vi "Read ERD Multiple Message Example.vi"(0 "GEA2 Reference In":refnum<k24>, 1 "Retry Count":i32=2, 2 "Read Timeout (ms)":u32=500, 5 "GEA Inputs":T3 {"Destination" format="%.0x"; "Source" format="%.0x"}, 11 "Error In":errorcluster, 12 "#ERDs per message":i32=1 min=1 step=1, 13 "Verify ERD Response?":bool=TRUE, 14 "Low Level Retry Count":u8=5 min=1 step=1) -> (4 "GEA2 Reference Out":refnum<k24>, 6 "Board ID":string, 8 "Raw Data Out":string[](array[string]), 15 "Error Out":errorcluster)   [LabVIEW 2016]
doc: "This is an example of how to use the GEA2 Read ERD multi-message VI. This VI splits up multiple ERD read requests into the number of messages you specify."
uses:
  Q:/Common/DLLs/GEA3/GeaCommunication.dll
  DLLs/GEA3/GeaCommunication.dll
  LabVIEW_GEA2_Toolkit.lvlibp/type defs/Source_Destination.ctl
  LabVIEW_GEA2_Toolkit.lvlibp/type defs/ERD Read Data In.ctl
  LabVIEW_GEA2_Toolkit.lvlibp/type defs/Data Type.ctl
  LabVIEW_GEA2_Toolkit.lvlibp
panel:
  in  "Read ERD List":T1[](array[typedef]) {"ERD Number" format="%.0x"}
  in  "Standalone?":bool=TRUE
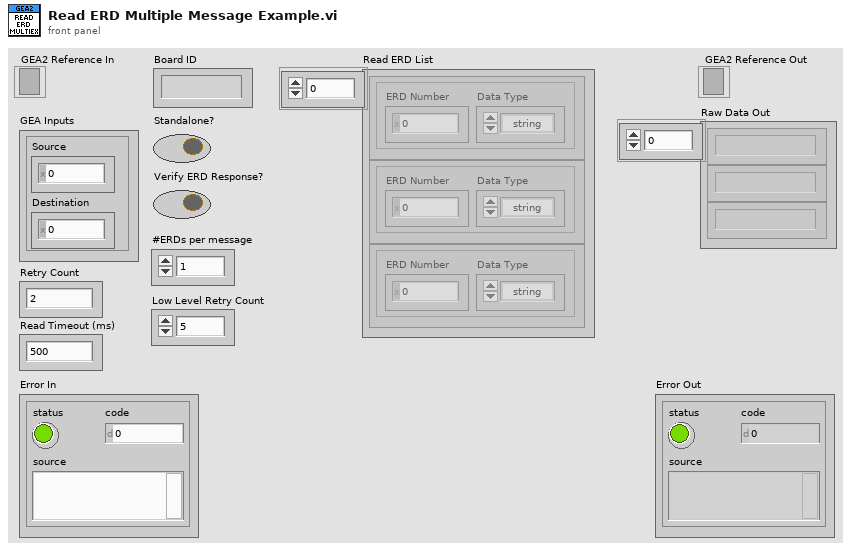
[diagram p1: front panel]
types:
  T1 = typedef "LabVIEW_GEA2_Toolkit.lvlibp/ERD Read Data In.ctl" = cluster{"ERD Number":u16, "Data Type":T2}
  T2 = typedef "LabVIEW_GEA2_Toolkit.lvlibp/Data Type.ctl" = enum16{"string", "boolean", "uint8_t", "uint16_t", "uint32_t", "uint64_t", "int8_t", "int16_t", "int32_t", "int64_t"}
  T3 = typedef "LabVIEW_GEA2_Toolkit.lvlibp/Source_Destination.ctl" = cluster{"Source":u8, "Destination":u8}
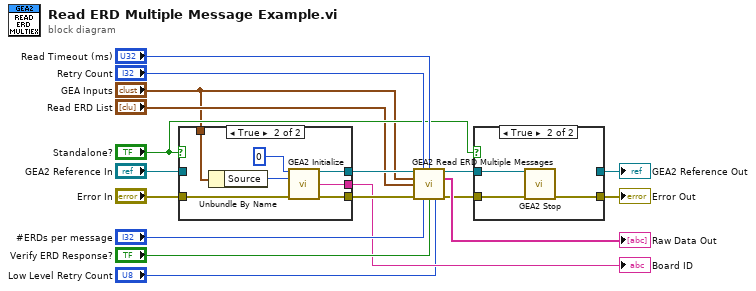
[diagram p0: block diagram]
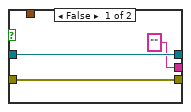
[diagram p3: hidden frame]
diagram:
  n1 = case shown="True" "Standalone?" {
    tunnel: [w20 w28] -> w15
    tunnel: "Error In" -> [w20 w27]
    tunnel: [w21 w25] -> w16
    tunnel: "GEA2 Reference In" -> [w21 _]
    tunnel: ["" ("Board ID") w24] -> w9
    tunnel: "GEA Inputs" -> [_ w23]
    frame False {
    }
    frame True {
      n2 = Unbundle By Name(w23) -> ("Source"=w22:u8)
      n3 = call "GEA2 Initialize.vi"("Board Index"=0, "Source Address"=w22, "error in"=w27) -> ("GEA2 Reference Out"=w25:refnum<k24>, "Board ID"=w24:string, "error out"=w28:errorcluster)  [unwired: 10 in]
    }
  }
  "Board ID" <- w9
  n4 = call "GEA2 Read ERD Multiple Messages.vi"("GEA2 Reference In"=w16, "Retry Count"="Retry Count", "Read Timeout (ms)"="Read Timeout (ms)", "GEA Inputs"="GEA Inputs", "Read ERD List"="Read ERD List", "Error In"=w15, "#ERDs per message"="#ERDs per message", "Verify ERD Response?"="Verify ERD Response?", "Low Level Retry Count"="Low Level Retry Count") -> ("GEA2 Reference Out"=w6:refnum<k24>, "Raw Data Out"=→"Raw Data Out":string[], "Error Out"=w7:errorcluster)  [unwired: 3 in, 1 out]
  n5 = case shown="True" "Standalone?" {
    tunnel: [w30 w33] -> w8
    tunnel: w7 -> [w30 w32]
    tunnel: w6 -> [w29 w31]
    tunnel: [w29 _] -> w5
    frame False {
    }
    frame True {
      n6 = call "GEA2 Stop.vi"("GEA2 Reference In"=w31, "Error In"=w32) -> ("Error Out"=w33:errorcluster)  [unwired: 13 in]
    }
  }
  "Error Out" <- w8
  "GEA2 Reference Out" <- w5
